vi "RewriteLoopsETC.vi"(1 "Type":enum16{"Tiny", "BotSpeak"}(ring), 2 "URAPI in":string) -> (0 "URAPI out":string)   [LabVIEW 2014]
panel:
  out "line #":i32[](array[numeric])
  out "labels":string[](array[string])
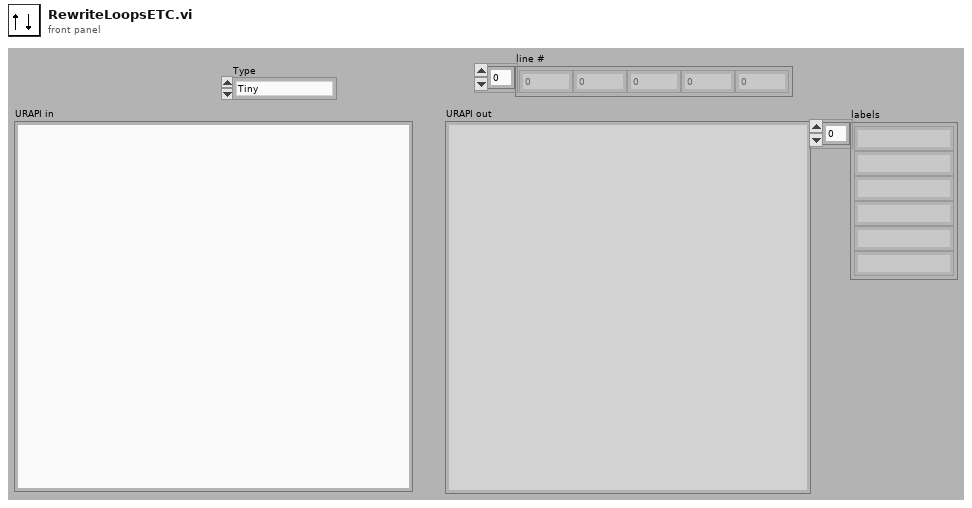
[diagram p1: front panel]
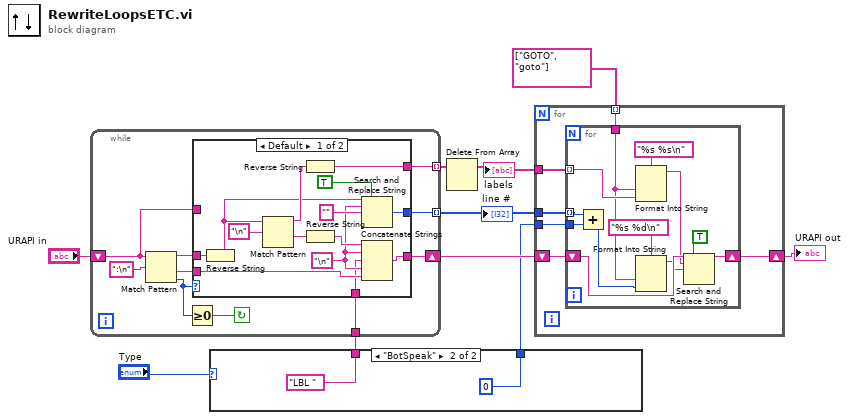
[diagram p0: block diagram]
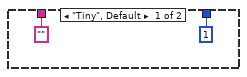
[diagram p2: hidden frame]
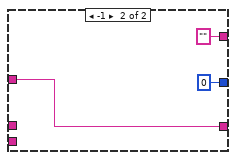
[diagram p3: hidden frame]
diagram:
  n1 = case shown="\"BotSpeak\"" "Type" {
    tunnel: ["" ("replace string (\"\")") "LBL " ("replace string (\"\")")] -> w3
    tunnel: [1 0] -> w2
    frame "Tiny", Default {
    }
    frame "BotSpeak" {
    }
  }
  n2 = while {
    shift-right: [w21] -> w7
    shift-left: "URAPI in" -> [w16]
    tunnel: [w20] -> w6 mode=indexing
    tunnel: [w19] -> w10 mode=indexing
    tunnel: w3 -> [w15]
    stop <- w23 continue-if-true
    n3 = Match Pattern(string=w16, regular expression=":\n") -> (before substring=w22:string, after substring=w18:string, offset past match=w17:i32)  [unwired: 1 in, 1 out]
    n4 = Greater Or Equal To 0?(x=w17) -> (x >= 0?=w23:bool)
    n5 = case shown="Default" w17 {
      tunnel: w22 -> [w38 _]
      tunnel: [w36 w39] -> w21
      tunnel: [w26 ""] -> w20
      tunnel: [w32 0 ("number of replacements")] -> w19
      tunnel: w18 -> [w29 _]
      tunnel: w16 -> [_ w39]
      tunnel: w15 -> [w25 _]
      frame Default {
        w27 = "\n" ("regular expression")
        n6 = Reverse String(1:w38) -> (0:w28:string)
        n7 = Match Pattern(string=w28, regular expression="\n") -> (before substring=w30:string, after substring=w31:string)  [unwired: 1 in, 2 out]
        n8 = Reverse String(1:w30) -> (0:w26:string)
        n9 = Reverse String(1:w31) -> (0:w33:string)
        n10 = Search and Replace String(replace all?=TRUE ("replace all? (F)"), input string=w28, search string=w27, replace string="" ("replace string (\"\")")) -> (number of replacements=w32:i32)  [unwired: 4 in, 3 out]
        n11 = Concatenate Strings(w33, w27, w25, w27, w29) -> (w36:string)
      }
      frame -1 {
      }
    }
  }
  "line #" <- w10
  n12 = Delete From Array(array=w6) -> (array with subset deleted=w5:string[])  [unwired: 2 in, 1 out]
  "labels" <- w5
  n13 = for {
    tunnel: w10 -> [w47]
    tunnel: w5 -> [w44]
    shift-right: [w46] -> w9
    shift-left: w7 -> [w45]
    tunnel: string[] ["GOTO", "goto"] -> [w43] mode=indexing
    tunnel: w2 -> [w42]
    n14 = for {
      shift-right: [w58] -> w46
      shift-left: w45 -> [w59]
      tunnel: w44 -> [w52] mode=indexing
      tunnel: w47 -> [w49] mode=indexing
      tunnel: w43 -> [w50]
      tunnel: w42 -> [w48]
      n15 = Add(x=w49, y=w48) -> (x+y=w55:i32)
      n16 = Format Into String(format string="%s %s\n" ("string"), w50, w52) -> (resulting string=w53:string)  [unwired: 2 in, 1 out]
      n17 = Format Into String(format string="%s %d\n" ("string"), w50, w55) -> (resulting string=w56:string)  [unwired: 2 in, 1 out]
      n18 = Search and Replace String(replace all?=TRUE ("replace all? (F)"), input string=w59, search string=w53, replace string=w56) -> (result string=w58:string)  [unwired: 4 in, 3 out]
    }
  }
  "URAPI out" <- w9
